vi "Sandbox VI 2.vi"() -> ()   [LabVIEW 2022 SP3]
doc: "The first bold characters are: 22, 23, 24, 25"
uses:
  <vilib>/Utility/traverseref.llb/TRef TravTarget.ctl
  <vilib>/Utility/traverseref.llb/VI Scripting - Traverse.lvlib
panel:
  out "# of Refs":i32
  out "error out":errorcluster
  out "Text":string
  out "Iteration":i32
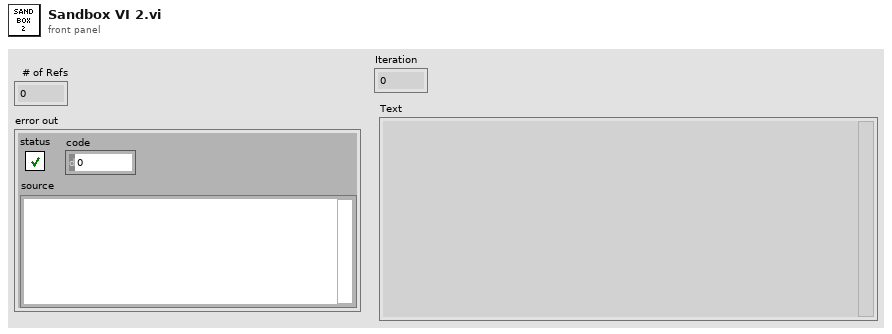
[diagram p1: front panel]
types:
  T1 = typedef "TRef TravTarget.ctl" = enum16{"FP", "BD", "Other"}
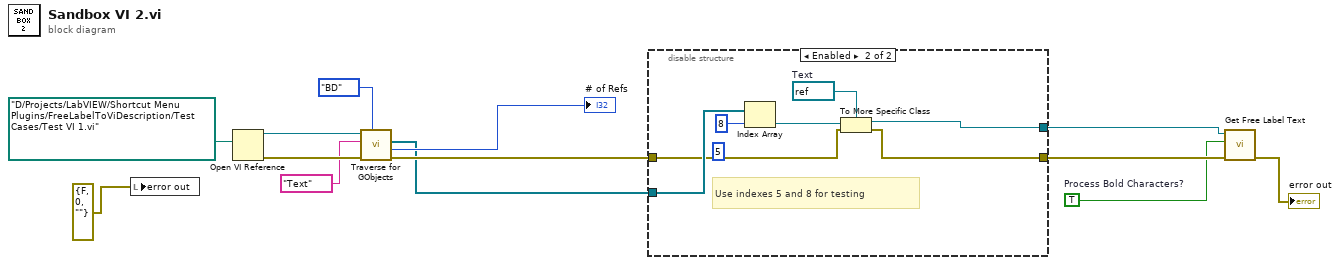
[diagram p0: block diagram]
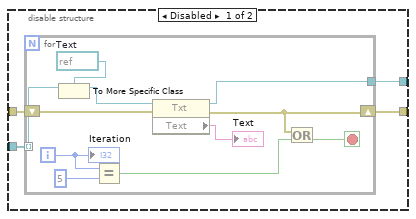
[diagram p2: hidden frame]
diagram:
  w1 = TRUE  # Process Bold Characters?
  n1 = local write "error out"(errorcluster {"status"=FALSE, "code"=0, "source"=""} ("error in (no error)")) -> ()
  n2 = Open VI Reference(vi path=path "D:/Projects/LabVIEW/Shortcut Menu Plugins/FreeLabelToViDescription/Test Cases/Test VI 1.vi") -> (vi reference=w11:refnum<vi>, error out=w12:errorcluster)  [unwired: 5 in]
  n3 = call <vilib>:"Traverse for GObjects.vi"("Traverse Target"=TRef_TravTarget."BD", "error in (no error)"=w12, "Class Name"="Text", "VI Refnum"=w11) -> ("error out"=w7:errorcluster, "# of Refs"=→"# of Refs":i32, "References"=w5:refnum<vi>[])  [unwired: 4 in, 1 out]
  n4 = disable-structure shown="Enabled" {
    disable-tunnel: w7 -> [w17 w32]
    disable-tunnel: [w16 w31] -> w3
    disable-tunnel: w5 -> [w15 w33]
    disable-tunnel: [w14 w29] -> w2
    frame Disabled {
      n5 = for {
        tunnel: w15 -> [w28] mode=indexing
        shift-right: [w23] -> w16
        shift-left: w17 -> [w25]
        tunnel: [w22] -> w14
        i -> [w20]
        stop <- w21 stop-if-true
        w26 = refnum<vi> refnum  # Text
        n6 = To More Specific Class(target class=w26, reference=w28) -> (specific class reference=w27:refnum<vi>)  [unwired: 1 in, 1 out]
        n7 = Equal?(x=w20, y=5) -> (x = y?=w18:bool)
        n8 = property class="Txt"(reference=w27, error in=w25) -> (reference out=w22:refnum<vi>, error out=w23:errorcluster, "Text"=→"Text":string)
        n9 = Or(x=w23, y=w18) -> (x .or. y?=w21:bool)
        "Iteration" <- w20
      }
    }
    frame Enabled {
      (unwired) 5 ("index")
      w30 = refnum<vi> refnum  # Text
      # "Use indexes 5 and 8 for testing"
      n10 = Index Array(array=w33, index=8) -> (element=w35:refnum<vi>)
      n11 = To More Specific Class(target class=w30, reference=w35, error in=w32) -> (specific class reference=w29:refnum<vi>, error out=w31:errorcluster)
    }
  }
  n12 = call "Get Free Label Text.vi"("Error In"=w3, "Process Bold Characters?"=w1, "Free Label Ref"=w2) -> ("Error Out"=→"error out":errorcluster)  [unwired: 6 in, 2 out]
